vi "Write Owning lib name.vi"(10 "Owning lib name":string, 11 "ProjectItem in":refnum<class "ProjectItem.lvclass">) -> (3 "ProjectItem out":refnum<class "ProjectItem.lvclass">)   [LabVIEW 2019, in "SolutionBuilder.lvlib" / "ProjectItem.lvclass"]
uses:
  ProjectItem.lvclass
  ProjectItem.lvclass/ProjectItem.ctl
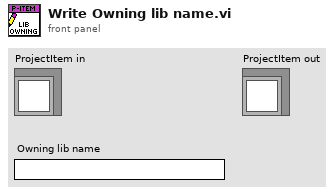
[diagram p1: front panel]
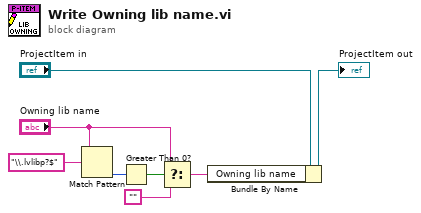
[diagram p0: block diagram]
diagram:
  n1 = Match Pattern(string="Owning lib name", regular expression="\\.lvlibp?$") -> (offset past match=w5:i32)  [unwired: 1 in, 3 out]
  n2 = Greater Than 0?(x=w5) -> (x > 0?=w4:bool)
  n3 = Select(t="Owning lib name", s=w4, f="") -> (s? t:f=w2:string)
  n4 = Bundle By Name(cluster="ProjectItem in", "Owning lib name"=w2) -> (→"ProjectItem out":refnum<class "ProjectItem.lvclass">)
